vi "Get Channel Status.vi"(5 "Channel":i32=1 min=1 max=2 step=1, 7 "Slave":i32=1 min=1 max=6 step=1, 8 "error in (no error)":errorcluster, 11 "VISA resource name":refnum<visa-resource-name>) -> (0 "error out":errorcluster, 2 "Channel Enabled":bool, 3 "VISA resource name out":refnum<visa-resource-name>)   [LabVIEW 2020, in "QuPMXdriver.lvlib"]
doc: "Returns status of channel."
uses:
  QuPMXdriver.lvlib
  <vilib>/ErrorRing/Error Ring.xnode
  <vilib>/Utility/error.llb/Error Cluster From Error Code.vi
panel:
  out "read buffer":string="SLV SL%d CH%d "
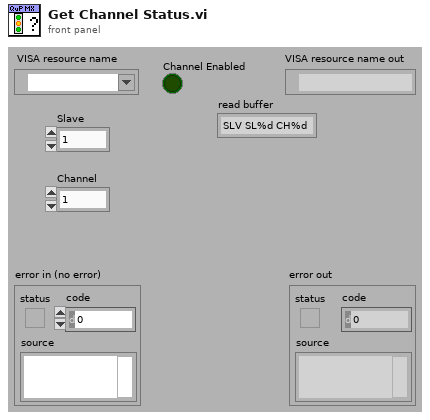
[diagram p1: front panel]
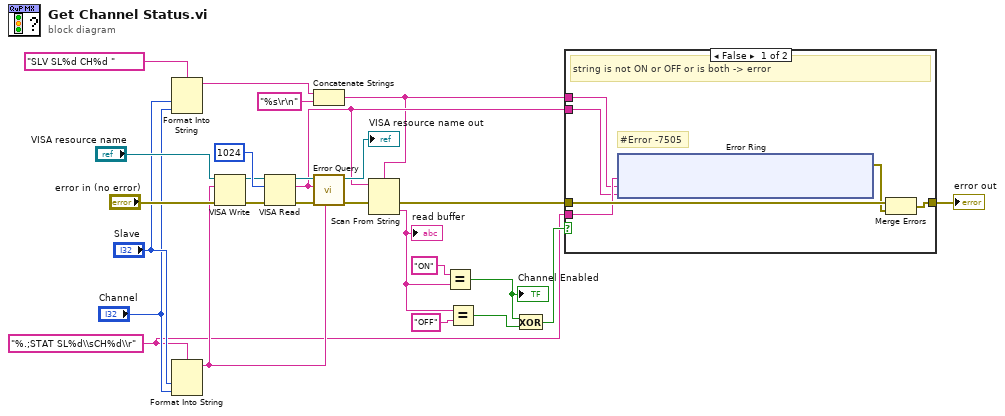
[diagram p0: block diagram]
diagram:
  w4 = "%.;STAT SL%d\\sCH%d\\r" ("format string")
  n1 = Format Into String(format string="SLV SL%d CH%d " ("read buffer"), "Slave", "Channel") -> (resulting string=w14:string)  [unwired: 2 in, 1 out]
  n2 = Format Into String(format string=w4, "Slave", "Channel") -> (resulting string=w19:string)  [unwired: 2 in, 1 out]
  n3 = VISA Write(VISA resource name="VISA resource name", write buffer=w19, error in (no error)="error in (no error)") -> (VISA resource name out=w21:refnum<visa-resource-name>, error out=w1:errorcluster)  [unwired: 1 out]
  n4 = VISA Read(VISA resource name=w21, byte count=u32 1024, error in (no error)=w1) -> (VISA resource name out=w22:refnum<visa-resource-name>, read buffer=w3:string, error out=w20:errorcluster)  [unwired: 1 out]
  n5 = Concatenate Strings(w14, "%s\r\n" ("read buffer")) -> (w2:string)
  n6 = call "Error Query.vi"("Last command"=w19, "error in (no error)"=w20, "Read buffer"=w3, "VISA resource name"=w22) -> ("error out"=w18:errorcluster, "VISA resource name out"=→"VISA resource name out":refnum<visa-resource-name>)  [unwired: 6 in]
  n7 = Scan From String(format string=w2, input string=w3, error in=w18) -> (error out=w6:errorcluster, output 1=w12:string)  [unwired: 2 in, 2 out]
  "read buffer" <- w12
  n8 = Equal?(x="ON", y=w12) -> (x = y?=w5:bool)
  "Channel Enabled" <- w5
  n9 = Equal?(x=w12, y="OFF") -> (x = y?=w9:bool)
  n10 = Exclusive Or(1:w9, 2:w5) -> (0:w8:bool)
  n11 = case shown="False" w8 {
    tunnel: [w31 w42] -> w7
    tunnel: w6 -> [w32 w42]
    tunnel: w4 -> [w29 _]
    tunnel: w3 -> [w28 _]
    tunnel: w2 -> [w27 _]
    frame False {
      # "#Error -7505"
      # "string is not ON or OFF or is both -> error"
      n12 = xnode "Error Ring"("parameter 0"=w29, "parameter 1"=w27, "parameter 2"=w28) -> ("error out"=w30:errorcluster)
      n13 = Merge Errors(w32, w30) -> (w31:errorcluster)
    }
    frame True {
    }
  }
  "error out" <- w7
